vi "_Read.vi"(8 "error in (no error)":errorcluster, 11 "Two Lockins in":refnum<class "Two Lockins.lvclass">) -> (0 "error out":errorcluster, 2 "X array":T1, 3 "Two Lockins out":refnum<class "Two Lockins.lvclass">)   [LabVIEW 2017, in "Two Lockins.lvclass"]
doc: "(Protected, Dynamic, Pure Virtual/Abstract) Perform a measurement and return one or more channels of data. Outsiders should not call this method, but instead the public \"Read Data.vi\"."
uses:
  Two Lockins.lvclass
  Utility Classes/Readable/X array.ctl
  Utility Classes/Readable/X.ctl
  Two Lockins.lvclass/Two Lockins.ctl
  Lockin/sr830/SR830.lvlib
  Utility Classes/Readable/Readable.lvclass
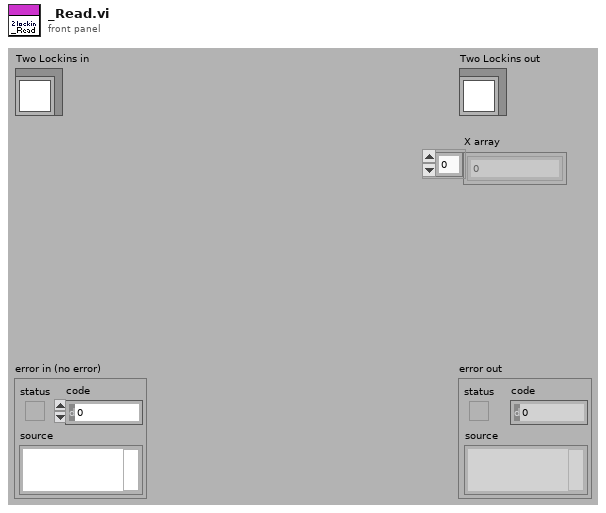
[diagram p1: front panel]
types:
  T1 = typedef "Readable.lvclass/X array.ctl" = T2[]
  T2 = typedef "Readable.lvclass/X.ctl" = dbl
  T3 = typedef "Lockin SR830.lvclass/Sensitivity.ctl" = u16
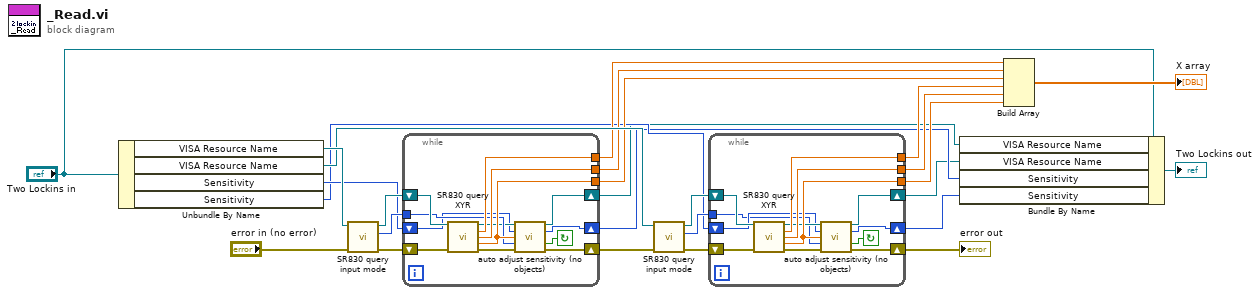
[diagram p0: block diagram]
diagram:
  n1 = Unbundle By Name("Two Lockins in") -> ("VISA Resource Name"=w26:refnum<visa-resource-name>, "VISA Resource Name"=w23:refnum<visa-resource-name>, "Sensitivity"=w18:T3, "Sensitivity"=w7:T3)
  n2 = call "SR830 query input mode.vi"("error in (no error)"="error in (no error)", "VISA resource name"=w26) -> ("error out"=w1:errorcluster, "input mode"=w25:enum16{"A", "A-B", "I (10^6)", "I (10^8)"}, "VISA resource name out"=w24:refnum<visa-resource-name>)  [unwired: 7 in]
  n3 = while {
    tunnel: w25 -> [w34]
    shift-right: [w27] -> w5
    shift-left: w18 -> [w28]
    shift-right: [w31] -> w13
    shift-left: w1 -> [w39]
    shift-right: [w29] -> w4
    shift-left: w24 -> [w38]
    tunnel: [w37] -> w22
    tunnel: [w36] -> w21
    tunnel: [w35] -> w20
    stop <- w32 continue-if-true
    n4 = call "SR830 query XYR.vi"("VISA resource name"=w38, "error in (no error)"=w39) -> ("VISA resource name out"=w30:refnum<visa-resource-name>, "X"=w37:dbl, "Y"=w36:dbl, "R"=w35:dbl, "error out"=w33:errorcluster)  [unwired: 9 in]
    n5 = call "auto adjust sensitivity (no objects).vi"("VISA Resource Name"=w30, "sensitivity"=w28, "R value"=w35, "Input Setting"=w34, "error in (no error)"=w33) -> ("VISA resource name out"=w29:refnum<visa-resource-name>, "sensitivity out"=w27:i8, "Repeat Measurement?"=w32:bool, "error out"=w31:errorcluster)  [unwired: 7 in]
  }
  n6 = call "SR830 query input mode.vi"("error in (no error)"=w13, "VISA resource name"=w23) -> ("error out"=w12:errorcluster, "input mode"=w14:enum16{"A", "A-B", "I (10^6)", "I (10^8)"}, "VISA resource name out"=w15:refnum<visa-resource-name>)  [unwired: 7 in]
  n7 = while {
    shift-right: [w41] -> w6
    shift-left: w7 -> [w42]
    shift-right: [w45] -> w11
    shift-left: w12 -> [w52]
    shift-right: [w43] -> w3
    shift-left: w15 -> [w51]
    tunnel: [w50] -> w10
    tunnel: [w49] -> w9
    tunnel: [w48] -> w8
    tunnel: w14 -> [w40]
    stop <- w46 continue-if-true
    n8 = call "SR830 query XYR.vi"("VISA resource name"=w51, "error in (no error)"=w52) -> ("VISA resource name out"=w44:refnum<visa-resource-name>, "X"=w50:dbl, "Y"=w49:dbl, "R"=w48:dbl, "error out"=w47:errorcluster)  [unwired: 9 in]
    n9 = call "auto adjust sensitivity (no objects).vi"("VISA Resource Name"=w44, "sensitivity"=w42, "R value"=w48, "Input Setting"=w40, "error in (no error)"=w47) -> ("VISA resource name out"=w43:refnum<visa-resource-name>, "sensitivity out"=w41:i8, "Repeat Measurement?"=w46:bool, "error out"=w45:errorcluster)  [unwired: 7 in]
  }
  "error out" <- w11
  n10 = Bundle By Name(cluster="Two Lockins in", "VISA Resource Name"=w4, "VISA Resource Name"=w3, "Sensitivity"=w5, "Sensitivity"=w6) -> (→"Two Lockins out":refnum<class "Two Lockins.lvclass">)
  n11 = Build Array(w22, w21, w20, w10, w9, w8) -> (→"X array":dbl[])
